vi "polarplot.vi"() -> ()   [LabVIEW 2016]
uses:
  <vilib>/Math Plots/3D Math Plots/3D Surface/3D Surface XCtrl/3D Surface.xctl
  <vilib>/Utility/file.llb/Read From Spreadsheet File (DBL).vi
  <vilib>/Math Plots/3D Math Plots/3D Surface/3D Surface Datatype/Public/Plot Helper (Vector).vi
  <vilib>/Math Plots/3D Math Plots/3D Surface/3D Surface Datatype/3D Surface Datatype.lvclass
panel:
  out "new picture":picture
  out "Angle (Degree)\nPolar":cluster{dbl, dbl}[](array[cluster]) caption="Power (dBm)\nPolar"
  out "3D Surface":refnum<class "3D Plot Datatype.lvclass">[](xcontrol)
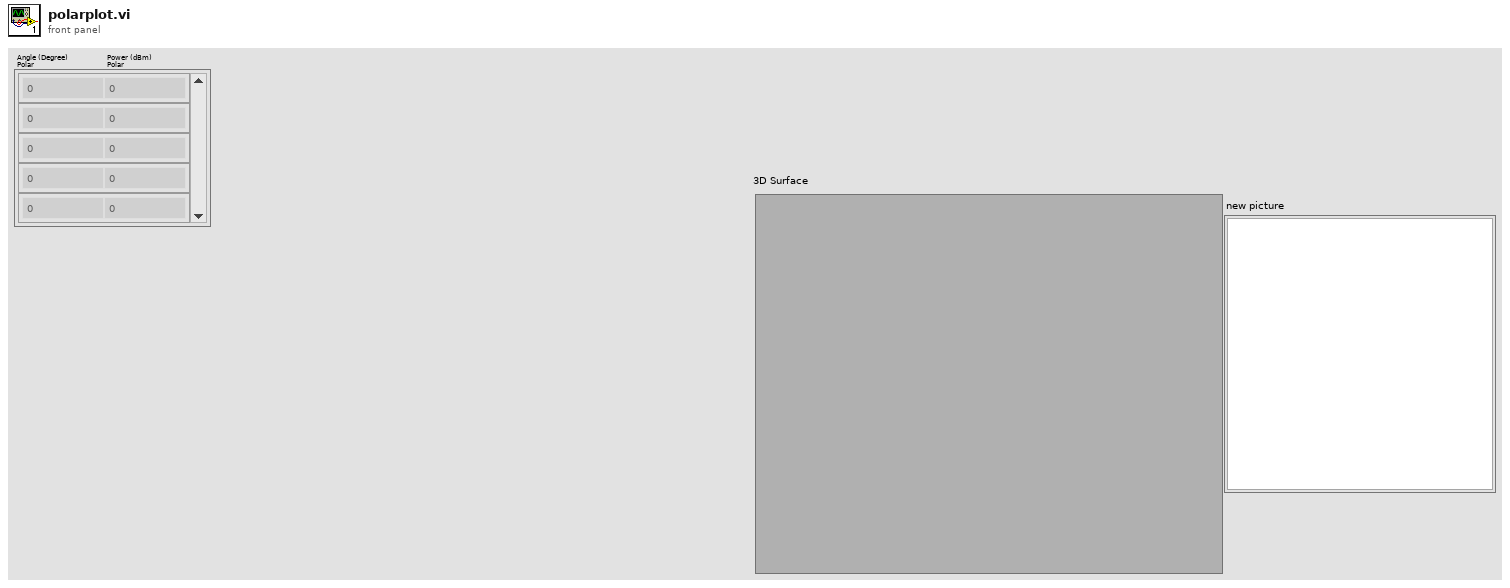
[diagram p1: front panel]
types:
  T1 = cluster{"maximum":dbl, "minimum":dbl, "clip to min":bool, "log?(F)":bool, "grid color":u32, "plot color":u32, "fmt and prec":cluster{"format":enum8{"Decimal", "Scientific", "Engineering", "Binary", "Octal", "Hex"}, "precision":u8}, "visible section":u16}
  T2 = cluster{"Font Name:":string, "Size":i16, "Strikeout?":bool, "Italic?":bool, "Underline?":bool, "Outline?":bool, "Shadow?":bool, "Bold?":bool}
  T3 = typedef "NI_Matrix.lvlib/RealMatrix.ctl" = dbl[][]
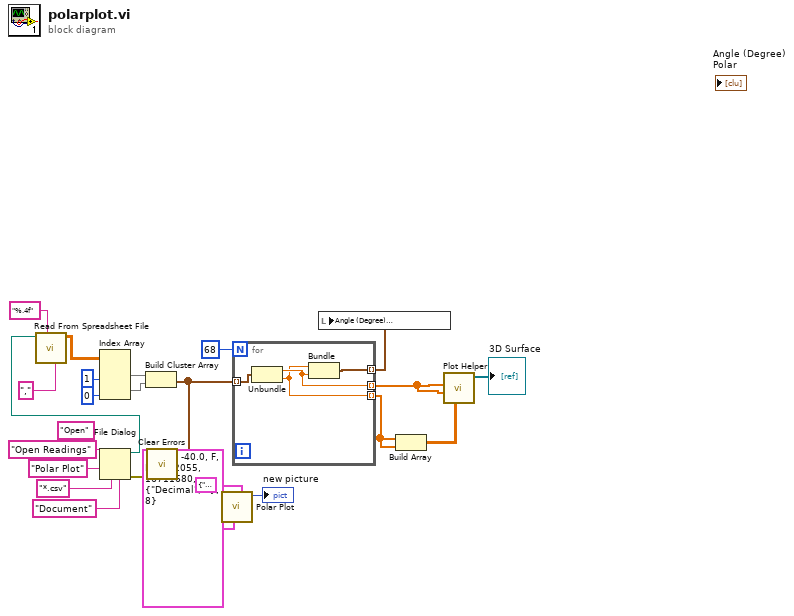
[diagram p0: block diagram]
diagram:
  (unwired) "Open" ("prompt")
  n1 = File Dialog(4:"Document" ("pattern (all files)"), 6:"*.csv" ("pattern (all files)"), 7:"Open Readings" ("prompt"), 9:"Polar Plot" ("default name")) -> (0:w6:errorcluster, 3:w5:path)  [unwired: 3 in, 2 out]
  n2 = call-poly <vilib>:"Read From Spreadsheet File.vi"("delimiter (\\t)"="," ("delimiter (\\t)"), "format (%.3f)"="%.4f", "file path (dialog if empty)"=w5) -> ("all rows"=w18:dbl[][])  [unwired: 4 in, 4 out]
  n3 = Index Array(array=w18, index (col) #1=1 ("disabled index (col)"), index (col) #2=0 ("index (col)")) -> (element #1=w20:dbl[], element #2=w19:dbl[])  [unwired: 2 in]
  n4 = Build Cluster Array(w20, w19) -> (w12:cluster{dbl, dbl}[])
  n5 = call <vilib>:"Clear Errors.vi"("error in (no error)"=w6) -> ()  [unwired: 5 in, 2 out]
  n6 = call <vilib>:"Polar Plot.vi"("[user-specified font]"=T2 {"Font Name:"="monaco", "Size"=9, "Strikeout?"=FALSE, "Italic?"=FALSE, "Underline?"=FALSE, "Outline?"=FALSE, "Shadow?"=FALSE, "Bold?"=TRUE}, "polar attributes"=T1 {"maximum"=-20.0, "minimum"=-40.0, "clip to min"=FALSE, "log?(F)"=FALSE, "grid color"=8882055, "plot color"=16711680, "fmt and prec"={"format"=enum."Decimal", "precision"=0}, "visible section"=8}, "data array [mag, phase (deg)]"=w12) -> ("new picture"=→"new picture":picture)  [unwired: 8 in]
  n7 = for {
    N: 68 -> [_]
    tunnel: w12 -> [w27] mode=indexing
    tunnel: [w26] -> w17 mode=indexing
    tunnel: [w25] -> w2 mode=indexing
    tunnel: [w24] -> w1 mode=indexing
    n8 = Unbundle(w27) -> (w25:dbl, w24:dbl)
    n9 = Bundle(w24, w25) -> (w26:cluster{dbl, dbl})  [unwired: 1 in]
  }
  n10 = local write "Angle (Degree)\nPolar"(w17) -> ()
  n11 = Build Array(w1, w1) -> (w3:T3)
  n12 = call-poly <vilib>:"Plot Helper.vi"("z matrix"=w3, "y vector"=w2, "x vector"=w2) -> ("3D Plot lvclass Array out"=→"3D Surface":refnum<class "3D Plot Datatype.lvclass">[])  [unwired: 3 in, 5 out]
